vi "DetectSqueezeRelease.vi"(4 "data in":dbl, 6 "ball in":timestamp, 7 "Now":timestamp, 9 "width squeeze in":u16, 10 "threshold release in":dbl, 11 "threshold squeeze in":dbl) -> (1 "Valley out":bool, 2 "Peak out":bool, 3 "to send?":bool)   [LabVIEW 2016]
doc: "checks if there was a squeeze /release in the past width pixels, and if passed enough\ntime since repviuosdetection (hardcoded 1 second). IMPORTANT: this has reentrant execution becasue otherwise doesn't detect peak when both hands squeeze together!"
uses:
  <vilib>/ptbypt/NI_PtbyPt.lvlib
panel:
  out "error":i32
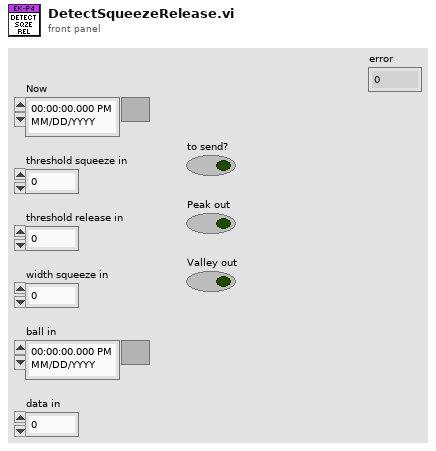
[diagram p1: front panel]
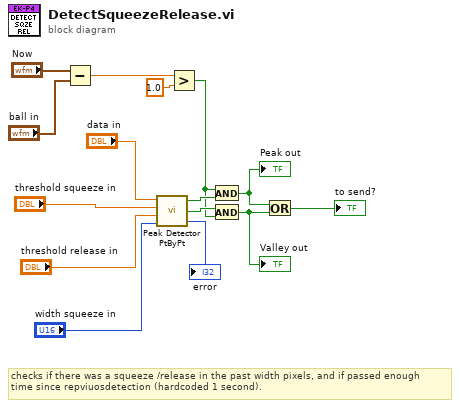
[diagram p0: block diagram]
diagram:
  # "checks if there was a squeeze /release in the past width pixels, and if passed enough\ntime since repviuosdetection (hardcoded 1 second)."
  n1 = Subtract(x="Now", y="ball in") -> (x-y=w12:dbl)
  n2 = call <vilib>:"Peak Detector PtByPt.vi"("x"="data in", "threshold peak"="threshold squeeze in", "threshold valley"="threshold release in", "width"="width squeeze in") -> ("peak"=w11:bool, "valley"=w10:bool, "error"=→"error":i32)  [unwired: 1 in]
  n3 = Greater?(x=w12, y=1.0) -> (0:w1:bool)
  n4 = And(x=w1, y=w11) -> (x .and. y?=w5:bool)
  "Peak out" <- w5
  n5 = And(x=w10, y=w1) -> (x .and. y?=w4:bool)
  "Valley out" <- w4
  n6 = Or(x=w5, y=w4) -> (x .or. y?=→"to send?":bool)
